vi "Determine Clicked Array Element Index.vi"(0 "reference":refnum<vi>, 2 "Coords of Click":T1) -> (4 "Clicked Index":i32[](array[numeric]), 6 "Clicked Row":i32, 8 "Clicked Col":i32, 10 "Vert Scroll Clicked?":bool, 14 "Index Display Clicked?":bool, 15 "Horizontal Scroll Clicked?":bool)   [LabVIEW 2014]
doc: "Determine Clicked Array Element Index.vi\n\n\nDescription:\nThis VI takes the coordinates of click input and determines the index of the array element that the user clicked.\n\nNOTE: Proper operation of the Determine Clicked Array Element Index VI requires that a caption has been created for the array of interest by following the numbered steps below:\n\n(1) Right click on the array of interest and select Visible Items >> Caption\n(The item should be checked)\n\n(2) Right click on the array of interest and select Visible Items >> Caption\n(The item should be un-checked)\n\n(3) Right click on the array of interest and select Visible Items >> Label\n(The item should be checked)\n\n(4) Save the VI\n\nInputs:\nArray Reference - Reference to the array to operate on.\n\nCoords of Click - The screen coordinates of the click within the array. These values are used to determine the index of the array element the user clicked.\n\nOutputs:\nClicked Index - The row and col indices of the item that the user clicked in the array.\n\nClicked Row - The row index of the item that the user clicked in the array.\n\nClicked Col - The column index of the item that the user clicked in the array.\n\nVert Scroll Clicked - Indicates if the vertical scrollbar was clicked.\n\nHorizontal Scroll Clicked - Indicates if the horizontal scrollbar was clicked.\n\nIndex Display Clicked - Indicates if the index display was clicked.\n\nDeveloped By:\nMark.ridgley\nMark.Ridgley_LabVIEW.Developer@comcast.net"
uses:
  <vilib>/Utility/miscctls.llb/LVPoint32TypeDef.ctl
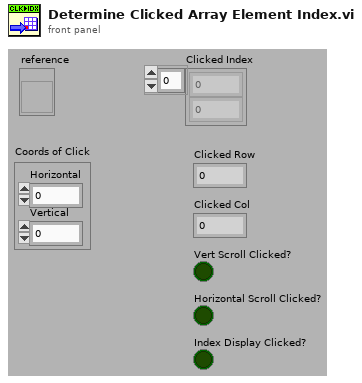
[diagram p1: front panel]
types:
  T1 = typedef "LVPoint32TypeDef.ctl" = cluster{"Horizontal":i32, "Vertical":i32}
  T2 = cluster{"Vertical Scrollbar Visible?":bool, "Vertical Scrollbar Left":i32, "Vertical Scrollbar Right":i32, "Vertical Scrollbar Clicked?":bool, "Horizontal Scrollbar Visible? ":bool, "Horizontal Scrollbar top":i32, "Horizontal Scrollbar Bottom":i32, "Horizontal Scrollbar Clicked?":bool}
  T3 = typedef "LVBoundsTypeDef.ctl" = cluster{"Width":u32, "Height":u32}
  T4 = typedef "LVPositionTypeDef.ctl" = cluster{"Left":i32, "Top":i32}
  T5 = cluster{"Number of Rows":u32, "Number of Columns":u32, "Column Width":u32, "Bounds":T3, "Position":T4, "Array Element.Position":T4, "Index Values":u32[], "Column Left Coordinates":i32[], "Row Top Coordinates":i32[], "Index Display Clicked?":bool, "Element Gap Displayed?":bool}
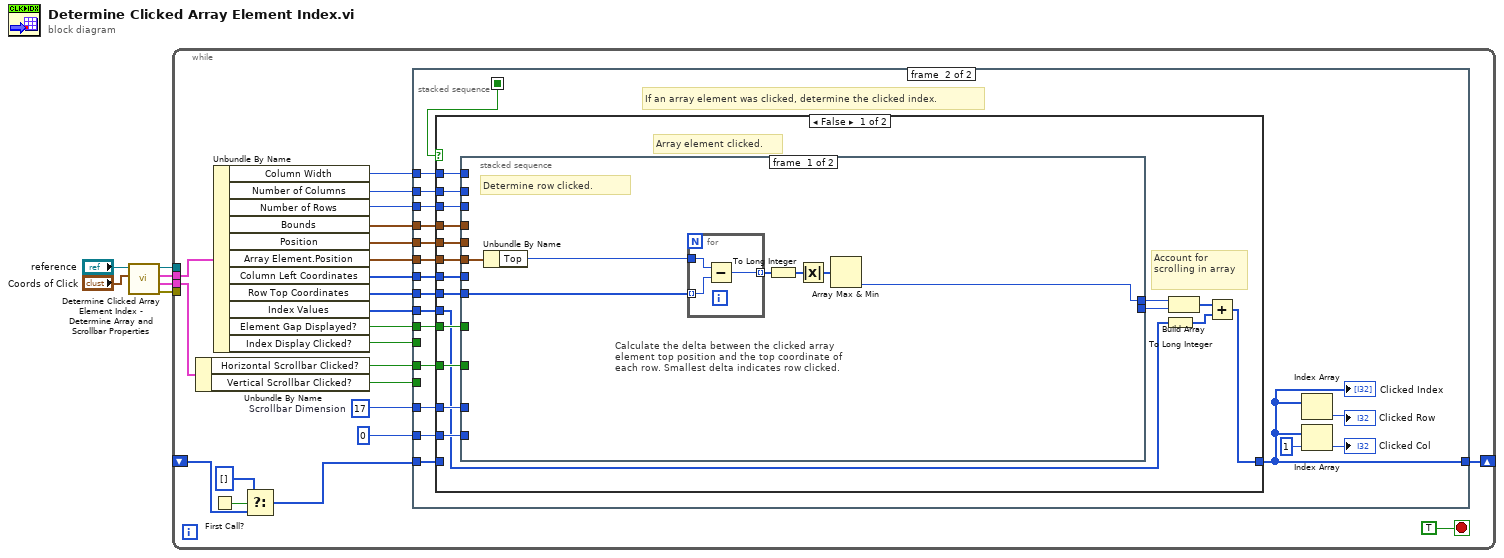
[diagram p0: block diagram]
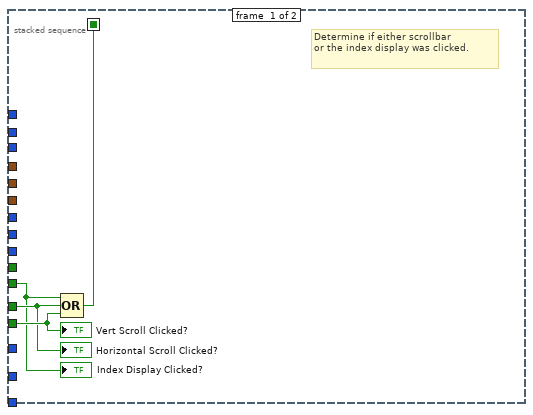
[diagram p2: hidden frame]
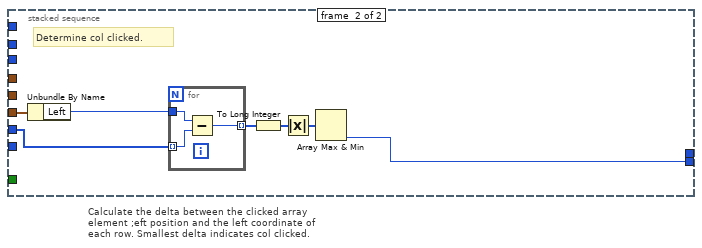
[diagram p3: hidden frame]
diagram:
  n1 = call "Determine Clicked Array Element Index - Determine Array and Scrollbar Properties.vi"("Coords of Click"="Coords of Click", "Array Reference"="reference") -> ("error out"=w4:errorcluster, "Scrollbar Properties"=w2:T2, "Array Properties"=w3:T5, "dup Array Reference"=w5:refnum<vi>)  [unwired: 6 in]
  n2 = while {
    shift-right: [w29] -> _
    shift-left: _ -> [w9]
    tunnel: w5 -> [_]
    tunnel: w4 -> [_]
    tunnel: w3 -> [w17]
    tunnel: w2 -> [w23]
    stop <- TRUE stop-if-true
    w27 = u32 17  # Scrollbar Dimension
    n3 = Unbundle By Name(w23) -> ("Horizontal Scrollbar Clicked?"=w22:bool, "Vertical Scrollbar Clicked?"=w18:bool)
    n4 = First Call?() -> (First Call?: T/F=w11:bool)
    n5 = Unbundle By Name(w17) -> ("Column Width"=w13:u32, "Number of Columns"=w19:u32, "Number of Rows"=w25:u32, "Bounds"=w24:T3, "Position"=w21:T4, "Array Element.Position"=w7:T4, "Column Left Coordinates"=w15:i32[], "Row Top Coordinates"=w16:i32[], "Index Values"=w20:u32[], "Element Gap Displayed?"=w12:bool, "Index Display Clicked?"=w14:bool)
    n6 = Select(t=i32[] [], s=w11, f=w9) -> (s? t:f=w8:i32[])
    n7 = stacked-sequence {
      seq-local: [w33 _] -> [_ w47]
      tunnel: [_ w42] -> w29
      tunnel: w8 -> [_ w50]
      tunnel: w20 -> [_ w49]
      tunnel: w7 -> [_ w48]
      tunnel: w24 -> [_ w46]
      tunnel: w21 -> [_ w45]
      tunnel: w22 -> [w31 w44]
      tunnel: w27 -> [_ w51]
      tunnel: u32 0 ("Number of Rows") -> [_ w52]
      tunnel: w19 -> [_ w39]
      tunnel: w25 -> [_ w38]
      tunnel: w18 -> [w32 _]
      tunnel: w16 -> [_ w37]
      tunnel: w15 -> [_ w36]
      tunnel: w14 -> [w30 _]
      tunnel: w13 -> [_ w35]
      tunnel: w12 -> [_ w34]
      frame #0 {
        # "Determine if either scrollbar\nor the index display was clicked."
        n8 = Compound Arithmetic op=OR(w30, w31, w32) -> (w33:bool)
        "Horizontal Scroll Clicked?" <- w31
        "Vert Scroll Clicked?" <- w32
        "Index Display Clicked?" <- w30
      }
      frame #1 {
        # "If an array element was clicked, determine the clicked index."
        n9 = case shown="False" w47 {
          tunnel: w48 -> [w68 _]
          tunnel: [w69 w91] -> w42
          tunnel: w50 -> [_ w91]
          tunnel: w49 -> [w53 _]
          tunnel: w46 -> [w67 _]
          tunnel: w45 -> [w66 _]
          tunnel: w44 -> [w65 _]
          tunnel: w51 -> [w63 _]
          tunnel: w52 -> [w62 _]
          tunnel: w39 -> [w59 _]
          tunnel: w38 -> [w58 _]
          tunnel: w37 -> [w57 _]
          tunnel: w36 -> [w56 _]
          tunnel: w35 -> [w55 _]
          tunnel: w34 -> [w54 _]
          frame False {
            # "Array element clicked."
            # "Account for scrolling in array"
            n10 = stacked-sequence {
              tunnel: [w73 _] -> w61
              tunnel: w66 -> [_ _]
              tunnel: w67 -> [_ _]
              tunnel: [_ w81] -> w60
              tunnel: w68 -> [w77 w87]
              tunnel: w63 -> [_ _]
              tunnel: w62 -> [_ _]
              tunnel: w65 -> [_ _]
              tunnel: w59 -> [_ _]
              tunnel: w58 -> [_ _]
              tunnel: w57 -> [w72 _]
              tunnel: w56 -> [_ w85]
              tunnel: w55 -> [_ _]
              tunnel: w54 -> [_ _]
              frame #0 {
                # "Determine row clicked."
                n11 = Unbundle By Name(w77) -> ("Top"=w76:i32)
                n12 = for "Calculate the delta between the clicked array element top position and the top coordinate of each row. Smallest delta indicates row clicked." {
                  tunnel: w72 -> [w79] mode=indexing
                  tunnel: w76 -> [w80]
                  tunnel: [w78] -> w75 mode=indexing
                  n13 = Subtract(x=w80, y=w79) -> (x-y=w78:i32)
                }
                n14 = To Long Integer(number=w75) -> (32bit integer=w71:i32[])
                n15 = Absolute Value(x=w71) -> (abs(x)=w74:i32[])
                n16 = Array Max & Min(array=w74) -> (min index (indices)=w73:i32)  [unwired: 3 out]
              }
              frame #1 {
                # "Determine col clicked."
                n17 = Unbundle By Name(w87) -> ("Left"=w84:i32)
                n18 = for "Calculate the delta between the clicked array element ;eft position and the left coordinate of each row. Smallest delta indicates col clicked." {
                  tunnel: w85 -> [w89] mode=indexing
                  tunnel: w84 -> [w90]
                  tunnel: [w88] -> w86 mode=indexing
                  n19 = Subtract(x=w90, y=w89) -> (x-y=w88:i32)
                }
                n20 = To Long Integer(number=w86) -> (32bit integer=w83:i32[])
                n21 = Absolute Value(x=w83) -> (abs(x)=w82:i32[])
                n22 = Array Max & Min(array=w82) -> (min index (indices)=w81:i32)  [unwired: 3 out]
              }
            }
            n23 = To Long Integer(number=w53) -> (32bit integer=w64:i32[])
            n24 = Build Array(w61, w60) -> (w70:i32[])
            n25 = Add(x=w70, y=w64) -> (x+y=w69:i32[])
          }
          frame True {
            # "Scrollbar or index display clicked. Do not update Clicked Index."
          }
        }
        "Clicked Index" <- w42
        n26 = Index Array(array=w42) -> (element=→"Clicked Row":i32)  [unwired: 1 in]
        n27 = Index Array(array=w42, index=1) -> (element=→"Clicked Col":i32)
      }
    }
  }
